vi "DualMotorControl_v0.vi"() -> ()   [LabVIEW 2019]
uses:
  <vilib>/myRIO/Common/Instrument Driver Framework/myRIO v1.0/Encoder/typedefs/Encoder Signal Mode.ctl
  <vilib>/myRIO/Instrument Drivers/Onboard IO/Encoder/typedefs/Encoder Reference.ctl
  <vilib>/myRIO/Common/Instrument Driver Framework/Utilities/typedefs/myRIO Generic Hardware Reference.ctl
  <vilib>/myRIO/Common/Instrument Driver Framework/Utilities/typedefs/Hardware Version Enum.ctl
  <vilib>/myRIO/Common/Instrument Driver Framework/Utilities/typedefs/myRIO v1.0 Reference.ctl
  <vilib>/myRIO/Common/Instrument Driver Framework/Utilities/typedefs/Generic FPGA Reference.ctl
  <vilib>/myRIO/Common/Instrument Driver Framework/myRIO v1.0/Encoder/typedefs/Encoder Channels Enum.ctl
  <vilib>/myRIO/Common/Instrument Driver Framework/myRIO v1.0/Encoder/typedefs/Encoder Configuration v1.0.ctl
  <vilib>/userDefined/High Color/nirio_resource_hc.ctl
  <vilib>/Platform/TimedLoop/XDataNode/timing_clust.ctl
  <vilib>/Platform/TimedLoop/XDataNode/nitl_modes.ctl
  <vilib>/Platform/TimedLoop/XDataNode/wakeup.ctl
  <vilib>/myRIO/Instrument Drivers/Onboard IO/PWM/typedefs/PWM Reference.ctl
  <vilib>/myRIO/Common/Instrument Driver Framework/myRIO v1.0/PWM/typedefs/PWM Channels Enum.ctl
  <vilib>/myRIO/Instrument Drivers/Onboard IO/PWM/typedefs/PWM Configuration.ctl
  <vilib>/myRIO/Instrument Drivers/Onboard IO/DIO/typedefs/DIO Reference.ctl
  <vilib>/myRIO/Common/Instrument Driver Framework/myRIO v1.0/DIO/typedefs/DIO Channels List.ctl
  <vilib>/myRIO/Common/Instrument Driver Framework/myRIO v1.0/DIO/typedefs/DIO Channels Enum.ctl
  <vilib>/myRIO/Common/Instrument Driver Framework/Utilities/vis/Is FPGA Ref Available.vi
  <vilib>/myRIO/Common/Instrument Driver Framework/myRIO v1.0/Encoder/vis/myRIO v1.1 Open Encoder.vi
  <vilib>/myRIO/Instrument Drivers/Onboard IO/Encoder/vis/Read.vi
  <vilib>/myRIO/Common/Instrument Driver Framework/myRIO v1.0/PWM/vis/myRIO v1.1 Open PWM.vi
  <vilib>/myRIO/Instrument Drivers/Onboard IO/PWM/vis/Set Duty Cycle and Frequency.vi
  <vilib>/myRIO/Common/Instrument Driver Framework/myRIO v1.0/DIO/vis/myRIO v1.1 Open DIO.vi
  <vilib>/myRIO/Instrument Drivers/Onboard IO/DIO/vis/Write.vi
  <vilib>/myRIO/Common/Instrument Driver Framework/Utilities/vis/Validate Channels.vi
  <vilib>/myRIO/Common/Instrument Driver Framework/myRIO v1.0/Encoder/vis/myRIO v1.0 Reserve Encoder.vi
  <vilib>/myRIO/Common/Instrument Driver Framework/myRIO v1.0/PWM/vis/myRIO v1.0 Reserve PWM.vi
  <vilib>/myRIO/Common/Instrument Driver Framework/myRIO v1.0/DIO/vis/myRIO v1.0 Reserve DIO.vi
  <vilib>/myRIO/Common/Instrument Driver Framework/myRIO v1.0/Encoder/vis/myRIO v1.0 Build MUX Configuration Encoder.vi
  <vilib>/myRIO/Common/Instrument Driver Framework/myRIO v1.0/Resource Manager/vis/myRIO v1.0 Reserve Channel List.vi
  <vilib>/myRIO/Common/Instrument Driver Framework/myRIO v1.0/PWM/vis/myRIO v1.0 Build MUX Configuration PWM.vi
  <vilib>/myRIO/Common/Instrument Driver Framework/myRIO v1.0/DIO/vis/myRIO v1.0 Build MUX Configuration DIO.vi
  <vilib>/myRIO/Common/Instrument Driver Framework/myRIO v1.0/Resource Manager/vis/myRIO v1.0 Create Configuration List.vi
  <vilib>/myRIO/Common/Instrument Driver Framework/myRIO v1.0/Resource Manager/vis/myRIO v1.0 Reserve Channel.vi
  <vilib>/myRIO/Common/Instrument Driver Framework/myRIO v1.0/Resource Manager/vis/myRIO v1.0 Unreserve Channel.vi
  <vilib>/myRIO/Common/Instrument Driver Framework/myRIO v1.0/Resource Manager/vis/myRIO v1.0 Build Mutex Name.vi
  <vilib>/Utility/VariantDataType/GetNumericInfo.vi
  <vilib>/Utility/error.llb/Error Cluster From Error Code.vi
  <vilib>/myRIO/Common/Instrument Driver Framework/myRIO v1.0/myRIO v1.1 Open.vi
  <vilib>/myRIO/Common/Instrument Driver Framework/Utilities/vis/IO Manager.vi
  <vilib>/myRIO/Common/Instrument Driver Framework/Utilities/vis/Configuration Manager.vi
  <vilib>/myRIO/Common/Instrument Driver Framework/myRIO v1.0/Resource Manager/vis/myRIO v1.0 Configure IO.vi
  <vilib>/myRIO/Common/Instrument Driver Framework/myRIO v1.0/myRIO v1.0 Close.vi
  <vilib>/myRIO/Common/Instrument Driver Framework/myRIO v1.0/Encoder/vis/myRIO v1.0 Configure Encoder.vi
  <vilib>/myRIO/Common/Instrument Driver Framework/myRIO v1.0/Encoder/vis/myRIO v1.0 Read Encoder.vi
  <vilib>/Instr/_visa.llb/VISA Configure Serial Port (Instr).vi
  <vilib>/myRIO/Common/Instrument Driver Framework/myRIO v1.0/PWM/vis/myRIO v1.0 Write PWM.vi
  <vilib>/myRIO/Common/Instrument Driver Framework/myRIO v1.0/DIO/vis/myRIO v1.0 Write DIO.vi
  <vilib>/Utility/file.llb/Write Delimited Spreadsheet (DBL).vi
  <vilib>/myRIO/Express VI/Onboard IO/Encoder/Encoder Express VI.xnode
  <vilib>/myRIO/Instrument Drivers/Onboard IO/Encoder/vis/myRIO Encoder Open.xnode
  <vilib>/myRIO/Common/Instrument Driver Framework/myRIO v1.0/Encoder/typedefs/Encoder Count Direction Enum.ctl
  <vilib>/platform/TimedLoop/XDataNode/XDataNode.xnode
  <vilib>/myRIO/Express VI/Onboard IO/PWM/PWM Express VI.xnode
  <vilib>/myRIO/Instrument Drivers/Onboard IO/PWM/vis/myRIO PWM Open.xnode
  <vilib>/myRIO/Express VI/Onboard IO/DO/DO Express VI.xnode
  <vilib>/myRIO/Instrument Drivers/Onboard IO/DIO/vis/myRIO DIO Open.xnode
  <vilib>/Platform/TimedLoop/XDataNode/XDNodeRunTimeDep.lvlib
  <vilib>/myRIO/Instrument Drivers/Onboard IO/Encoder/Encoder.lvlib
  <vilib>/myRIO/Instrument Drivers/Onboard IO/DIO/DIO.lvlib
  <vilib>/myRIO/Instrument Drivers/Onboard IO/PWM/PWM.lvlib
panel:
  out "DC Velocity Graph":cluster{dbl[], dbl[]}[](graph)
  out "DC Position Graph":cluster{dbl[], dbl[]}[](graph)
  out "DC Velocity Chart":cluster{dbl, dbl}(graph)
  out "Duty cycle":dbl(graph)
  out "Duty cycle":dbl
  in  "Frequency":dbl=1000.0
  in  "Gain":T1={"P Gain"=0.5, "I Gain"=0.0, "D Gain"=0.005}
  out "DC Position Chart":cluster{dbl, dbl}(graph)
  in  "Encoder_Count":dbl=54991.0
  in  "t_shift":dbl=0.000125
  in  "T_ratio":dbl=10.0
  in  "buffer ratio":dbl=0.3
  in  "first or second tripod":bool
  in  "data of 5th order formula\nts,tair,a1-a6":dbl[](array[numeric])
  in  "format (%.3f)":string="%.3f"
  in  "file path (dialog if empty)":path
  out "error out":errorcluster
  in  "baud rate (9600)":u32=500000
  in  "VISA resource name":refnum<visa-resource-name>="ASRL2::INSTR"
  in  "stop":bool
  in  "const posotion":dbl=180.0
  out "write to visa":string
  out "read from visa":string
  out "sine position":dbl
  out "time":dbl
  out "iteration":i32
  in  "const(f)/sine(t)":bool
  in  "graph plot freq.":i32=1
  out "Servo Position Graph":cluster{dbl[], dbl[]}[](graph)
  in  "sinewave period":dbl=10.0
  in  "Loop Period":i64=5
  # "Servo motor"
  # "Read data to csv file"
  # "Read data to csv file"
  # "visa setting"
  # "servo setting"
  # "Timed loop status"
  # "DC motor"
  # "R-SLIP Parameters"
  # "v = 1; a = 15"
  # "v = 1.25; a = 15"
  # "v = 1.5; a = 15"
  # "0.184067181524967\n0.263820978418769\n256152.551336786\n-30272.30000274\n-9876.03760433421\n-1096.38594197941\n885.91817900106\n-44.6781799901984"
  # "0.215241998794118\n0.254514142390288\n4771.41078363533\n62185.8763006578\n-22508.5336527453\n390.805502041188\n686.695311017595\n-40.4128145310291"
  # "0.163616269216122\n0.27489641502463\n771965.39318528\n-201617.027694185\n8828.08396944145\n-2683.04589908678\n1085.57303422127\n-48.5860395324432"
  # "v = 1.75; a = 15"
  # "v = 2; a = 15"
  # "v = 2.25; a = 15"
  # "0.148651048423414\n0.288542414074344\n1776973.44893281\n-511591.467559457\n38775.9830765103\n-4576.94506688942\n1289.39828252671\n-52.3115561007577"
  # "0.136976185169818\n0.304016701267508\n3461279.85083822\n-993110.73746345\n80544.6579529191\n-6699.48295844177\n1494.82265451498\n-55.8934424469099"
  # "0.134381902205816\n0.369022171779704\n3272804.8365432\n-899365.569589567\n71225.2463409934\n-7039.10791102172\n1512.66147498591\n-59.3408899720725"
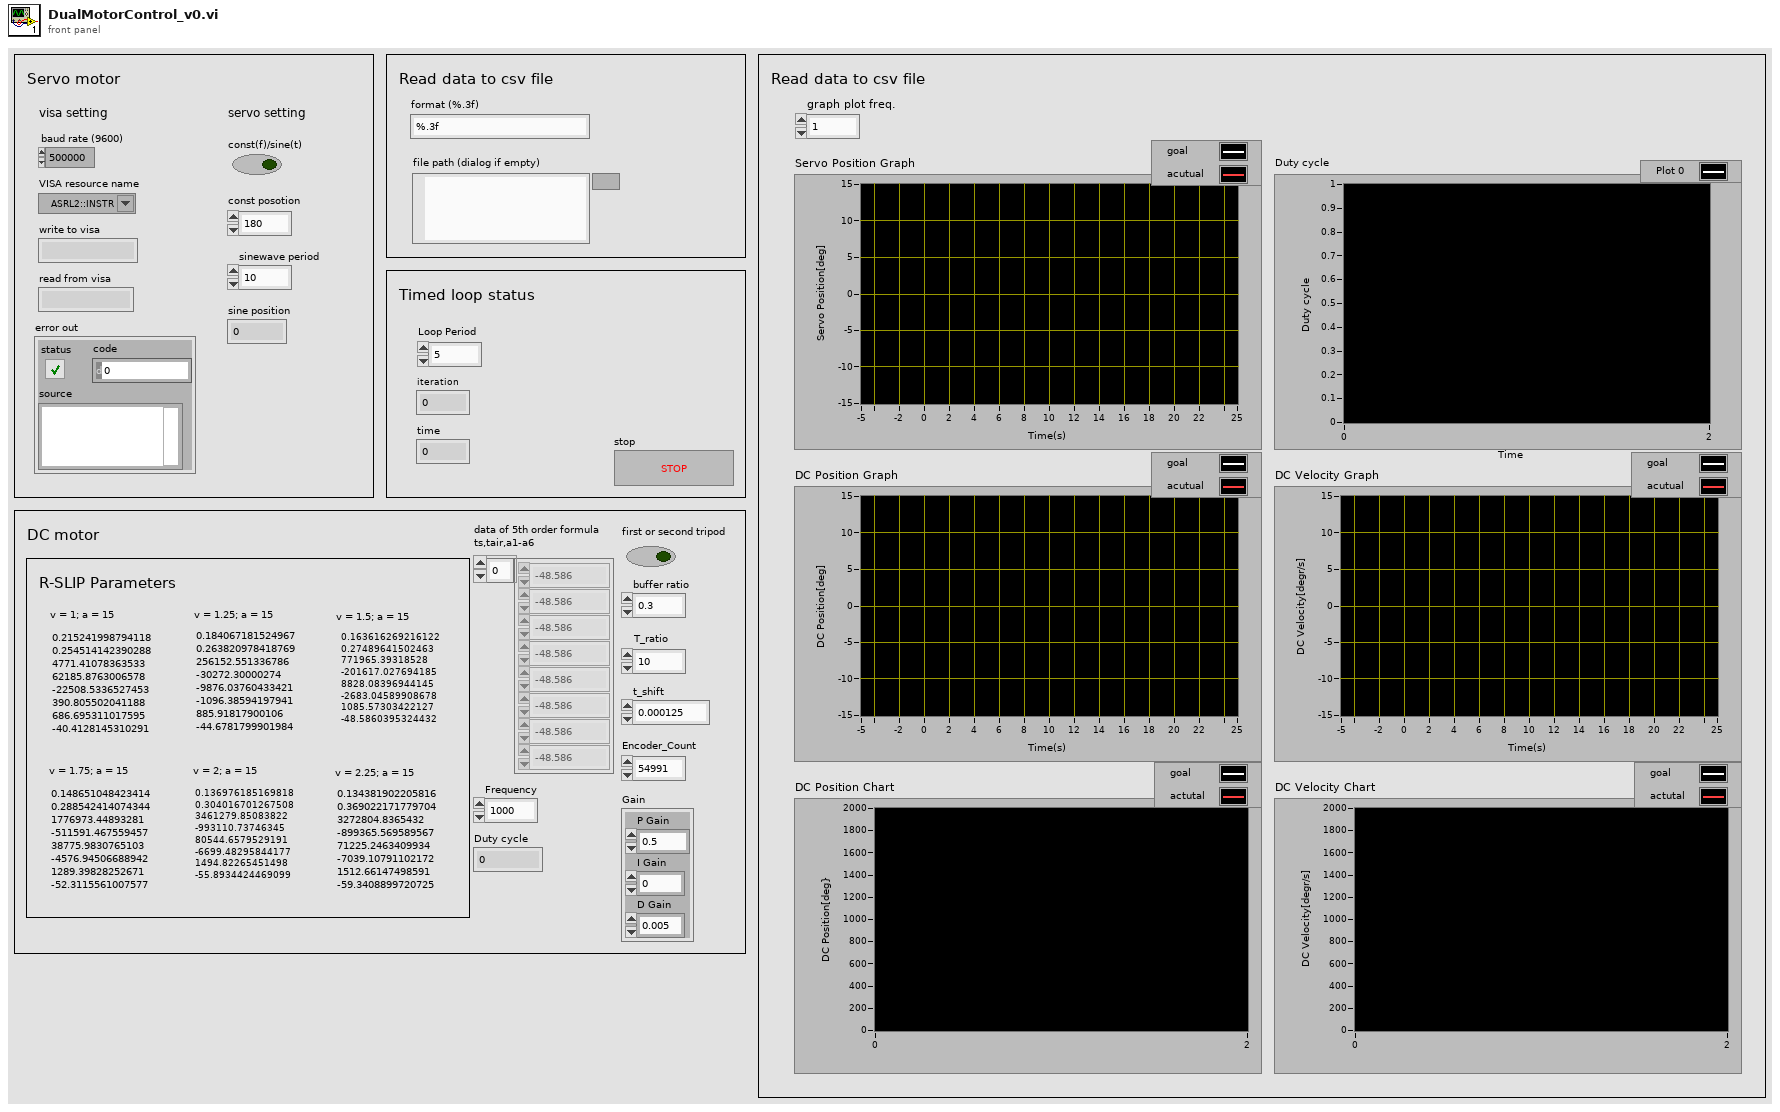
[diagram p1: front panel]
types:
  T1 = cluster{"P Gain":dbl, "I Gain":dbl, "D Gain":dbl}
  T2 = typedef "Encoder.lvlib/Encoder Reference.ctl" = cluster{"myRIO Reference":T3, "Encoder Channels Enum":T7}
  T3 = typedef "myRIO Generic Hardware Reference.ctl" = cluster{"myRIO Model":T4, "myRIO Hardware Reference":T5}
  T4 = typedef "Hardware Version Enum.ctl" = enum16{"Unknown", "myRIO-1900", "myRIO-1950", "roboRIO", "NI ELVIS RIO CM", "ELVIS III"}
  T5 = typedef "myRIO v1.0 Reference.ctl" = cluster{"Generic FPGA Reference":T6, "Allow multiple opens":bool}
  T6 = typedef "Generic FPGA Reference.ctl" = refnum<k20>
  T7 = typedef "Encoder Channels Enum.ctl" = enum16{"Not Connected", "C/ENC0", "C/ENC1", "A/ENC", "A/ENC0", "A/ENC1", "A/ENC2", "A/ENC3", "A/ENC4", "A/ENC5", "A/ENC6", "A/ENC7", "A/ENC8", "A/ENC9", "B/ENC", "B/ENC0", "B/ENC1", "B/ENC2", "B/ENC3", "B/ENC4", "B/ENC5", "B/ENC6", "B/ENC7", "B/ENC8", "B/ENC9", "DIO/ENC0", "DIO/ENC1", "DIO/ENC2", "DIO/ENC3", "DIO/ENC4"}
  T8 = typedef "Encoder Signal Mode.ctl" = enum16{"Quadrature phase signal", "Step and direction signal"}
  T9 = typedef "nirio_resource_hc.ctl" = tag
  T10 = cluster{"set position":dbl, "set position":dbl, "set position":dbl, "set position":dbl, "set position":dbl, "set position":dbl}
  T11 = typedef "DIO.lvlib/DIO Reference.ctl" = cluster{"myRIO Reference":T3, "DIO Channels List":T12}
  T12 = typedef "DIO Channels List.ctl" = T13[]
  T13 = typedef "DIO Channels Enum.ctl" = enum16{"Not Connected", "C/DIO0", "C/DIO1", "C/DIO2", "C/DIO3", "C/DIO4", "C/DIO5", "C/DIO6", "C/DIO7", "A/DIO0", "A/DIO1", "A/DIO2", "A/DIO3", "A/DIO4", "A/DIO5", "A/DIO6", "A/DIO7", "A/DIO8", "A/DIO9", "A/DIO10", "A/DIO11", "A/DIO12", "A/DIO13", "A/DIO14", "A/DIO15", "A/DIO16", "A/DIO17", "A/DIO18", "A/DIO19", "B/DIO0", "B/DIO1", "B/DIO2", "B/DIO3", "B/DIO4", "B/DIO5", "B/DIO6", "B/DIO7", "B/DIO8", "B/DIO9", "B/DIO10", "B/DIO11", "B/DIO12", "B/DIO13", "B/DIO14", "B/DIO15", "B/DIO16", "B/DIO17", "B/DIO18", "B/DIO19", "LED0", "LED1", "LED2", "LED3", "Button0", "DIO/DIO0", "DIO/DIO1", "DIO/DIO2", "DIO/DIO3", "DIO/DIO4", "DIO/DIO5", "DIO/DIO6", "DIO/DIO7", "DIO/DIO8", "DIO/DIO9", "SPI/CS0", "SPI/CS1", "SPI/CS2", "SPI/CS3", "LED RADIO (Green)", "LED RADIO (Red)", "LED COMM (Green)", "LED COMM (Red)", "LED MODE (Green)", "LED MODE (Red)"}
  T14 = typedef "PWM.lvlib/PWM Reference.ctl" = cluster{"myRIO Reference":T3, "PWM Channels Enum":T15, "PWM Configuration":T16}
  T15 = typedef "PWM Channels Enum.ctl" = enum16{"Not Connected", "C/PWM0", "C/PWM1", "A/PWM0", "A/PWM1", "A/PWM2", "A/PWM3", "A/PWM4", "A/PWM5", "A/PWM6", "A/PWM7", "A/PWM8", "A/PWM9", "A/PWM10", "A/PWM11", "A/PWM12", "A/PWM13", "A/PWM14", "A/PWM15", "A/PWM16", "A/PWM17", "A/PWM18", "A/PWM19", "B/PWM0", "B/PWM1", "B/PWM2", "B/PWM3", "B/PWM4", "B/PWM5", "B/PWM6", "B/PWM7", "B/PWM8", "B/PWM9", "B/PWM10", "B/PWM11", "B/PWM12", "B/PWM13", "B/PWM14", "B/PWM15", "B/PWM16", "B/PWM17", "B/PWM18", "B/PWM19", "PWM/PWM0", "PWM/PWM1", "PWM/PWM2", "PWM/PWM3", "PWM/PWM4", "PWM/PWM5", "PWM/PWM6", "PWM/PWM7", "PWM/PWM8", "PWM/PWM9"}
  T16 = typedef "PWM.lvlib/PWM Configuration.ctl" = cluster{"Frequency":dbl, "Duty Cycle":dbl}
  T17 = typedef "XDNodeRunTimeDep.lvlib/timing_clust.ctl" = cluster{"Expected End [f-1]":u64, "Actual End [f-1]":u64, "Finished Late? [f-1]":bool, "Expected End [i-1]":u64, "Actual End [i-1]":u64, "Finished Late? [i-1]":bool, "Expected Start [i]":u64, "Actual Start [i]":u64, "Expected Start [f]":u64, "Actual Start [f]":u64, "Source Name":string, "Structure Name":string, "Period":i64, "Deadline":i64, "Offset":i64, "Start":i64, "Priority":i32, "Timeout":i32, "Mode":T18, "Wakeup Reason":T19, "Error":errorcluster, "Source Type":string, "Secondary Source Type":string, "Global End Time":u64, "Global Start Time":u64, "Frame Duration":u64, "Iteration Duration":u64, "Assigned CPU":i32, "I/O Scan Engine Mode":u32}
  T18 = typedef "XDNodeRunTimeDep.lvlib/nitl_modes.ctl" = enum32{"No Change", "Process missed periods, maintain original phase", "Discard missed periods, maintain original phase", "Process missed periods, ignore original phase", "Discard missed periods, ignore original phase"}
  T19 = typedef "XDNodeRunTimeDep.lvlib/wakeup.ctl" = enum32{"Normal", "Aborted", "Asynchronous wakeup", "Timing source error", "Timed loop error", "Timeout"}
  T20 = cluster{"[0]":dbl, "[1]":dbl, "[2]":dbl, "[3]":dbl, "[4]":dbl, "[5]":dbl}
  T21 = cluster{"set position":i32, "set position":i32, "set position":i32, "set position":i32, "set position":i32, "set position":i32}
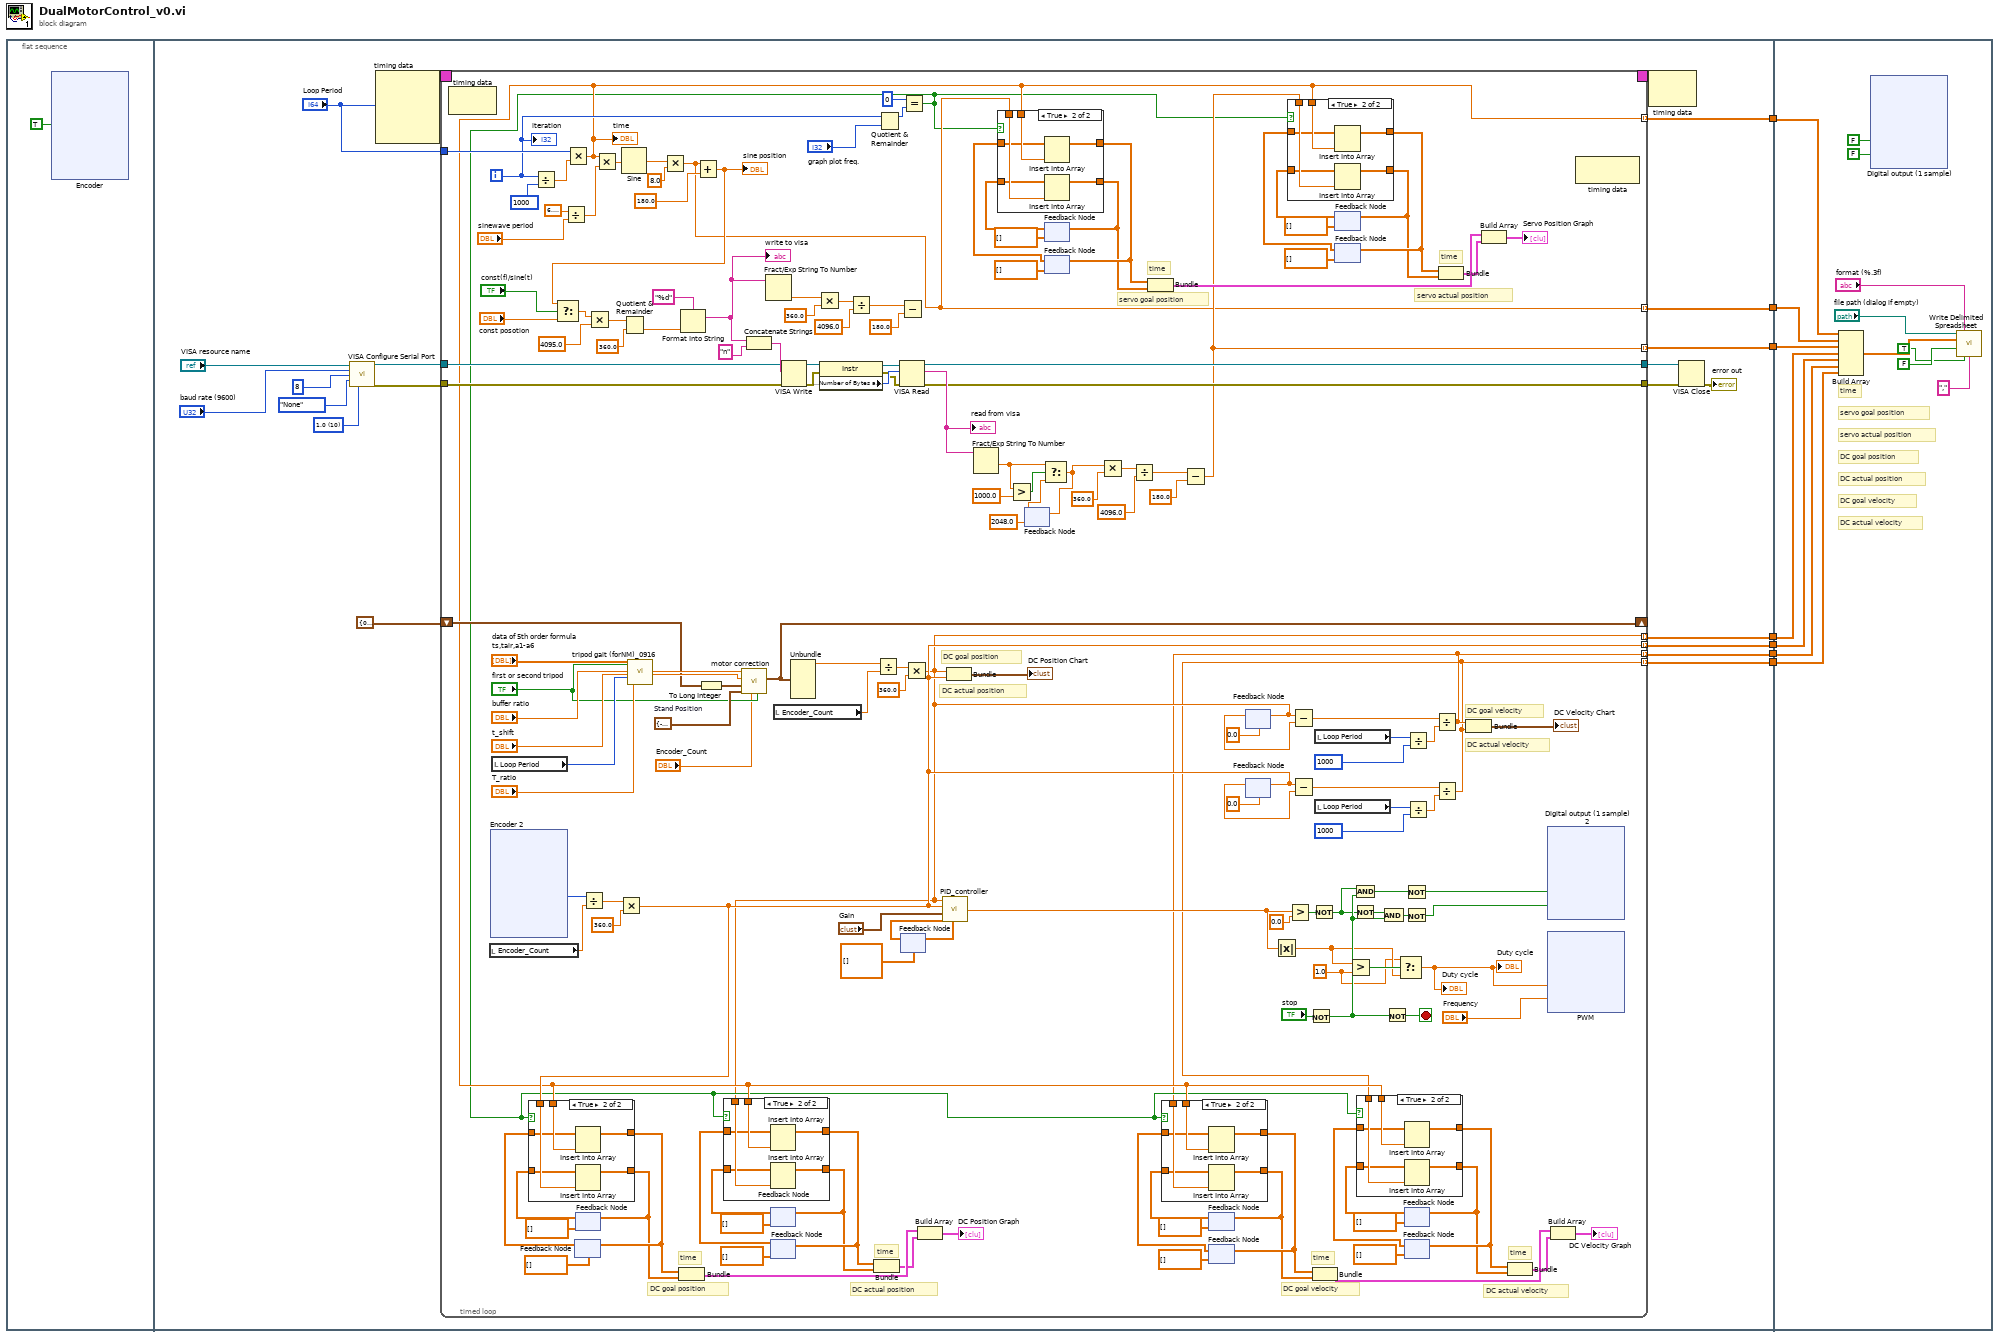
[diagram p0: block diagram]
diagram:
  n1 = flat-sequence {
    tunnel: [w63] -> w7
    tunnel: [w62] -> w6
    tunnel: [w61] -> w5
    tunnel: [w59] -> w4
    tunnel: [w58] -> w3
    tunnel: [w57] -> w2
    tunnel: [w56] -> w1
    tunnel: w7 -> [w414]
    tunnel: w6 -> [w413]
    tunnel: w5 -> [w415]
    tunnel: w4 -> [w412]
    tunnel: w3 -> [w411]
    tunnel: w2 -> [w410]
    tunnel: w1 -> [w409]
    frame #0 {
      n2 = xnode "Encoder"("Reset Counter"=TRUE) -> ()  [unwired: 1 in, 4 out]
    }
    frame #1 {
      w70 = u16 10 items=["1.0"=10, "1.5"=15, "2.0"=20] ("stop bits (10: 1 bit)")
      n3 = call-poly "VISA Configure Serial Port"("VISA resource name"="VISA resource name", "baud rate (9600)"="baud rate (9600)", "data bits (8)"=u16 8, "parity (0:none)"=enum16{"None", "Odd", "Even", "Mark", "Space"}."None", "stop bits (10: 1 bit)"=w70) -> ("VISA resource name out"=w69:refnum<visa-resource-name>, "error out"=w68:errorcluster)  [unwired: 9 in]
      n4 = node-c288("Loop Period") -> (w75:T17)  [unwired: 3 in]
      n5 = timed-loop {
        timing: w75 -> [_]
        timing-out: [_] -> w74
        tunnel: "Loop Period" -> [w184]
        tunnel: w68 -> [w185]
        tunnel: [w182] -> w67
        tunnel: w69 -> [w186]
        tunnel: [w181] -> w60
        tunnel: [w99] -> w63 mode=indexing
        tunnel: [w180] -> w62 mode=indexing
        tunnel: [w80] -> w61 mode=indexing
        shift-right: [w161] -> _
        shift-left: T10 {"set position"=0.0, "set position"=0.0, "set position"=0.0, "set position"=0.0, "set position"=0.0, "set position"=0.0} ("Setpoint_to_motor") -> [w162]
        tunnel: [w78] -> w59 mode=indexing
        tunnel: [w96] -> w58 mode=indexing
        tunnel: [w77] -> w57 mode=indexing
        tunnel: [w76] -> w56 mode=indexing
        i -> [w183]
        stop <- w131 stop-if-true
        w128 = 1.0 ("y")
        w160 = T20 {"[0]"=-27495.5, "[1]"=-27495.5, "[2]"=-27495.5, "[3]"=-27495.5, "[4]"=-27495.5, "[5]"=-27495.5}  # Stand Position
        # "time"
        # "DC actual velocity"
        # "time"
        # "DC goal velocity"
        # "time"
        # "DC actual position"
        # "time"
        # "DC goal position"
        # "DC actual velocity"
        # "DC goal velocity"
        # "DC actual position"
        # "DC goal position"
        # "time"
        # "servo actual position"
        # "time"
        # "servo goal position"
        n6 = node-c288() -> ()  [unwired: 1 in, 1 out]
        n7 = local read "Encoder_Count"() -> (w153:dbl)
        n8 = xnode "Encoder 2"() -> ("Counter Value"=w152:i32)  [unwired: 2 in, 3 out]
        n9 = local read "Loop Period"() -> (w167:i64)
        n10 = Divide(x=w183, y=i64 1000) -> (x/y=w216:dbl)
        n11 = Divide(x=6.283185307179586, y="sinewave period") -> (x/y=w171:dbl)
        n12 = Multiply(x=w184, y=w216) -> (x*y=w80:dbl)
        "time" <- w80
        n13 = feedback #1(dbl[] []) -> (w111:dbl[])
        n14 = feedback #2(dbl[] []) -> (w114:dbl[])
        n15 = Divide(x=w152, y=w153) -> (x/y=w150:dbl)
        n16 = Multiply(x=w80, y=w171) -> (x*y=w219:dbl)
        n17 = Multiply(x=w150, y=360.0 ("x")) -> (x*y=w96:dbl)
        n18 = Sine(x=w219) -> (sin(x)=w204:dbl)
        n19 = call "tripod gait (forNM)_0916.vi"("data of 5th order formula\nts,tair,a1-a6"="data of 5th order formula\nts,tair,a1-a6", "first or second"="first or second tripod", "buffer ratio"="buffer ratio", "t_shift"="t_shift", "sample time"=w167, "T_ratio"="T_ratio") -> ("Set Point"=w165:dbl, "Set Point 2"=w164:dbl)  [unwired: 4 in, 16 out]
        n20 = Multiply(x=w204, y=8.0) -> (x*y=w99:dbl)
        n21 = Add(x=w99, y=180.0) -> (x+y=w214:dbl)
        "sine position" <- w214
        n22 = Select(t=w214, s="const(f)/sine(t)", f="const posotion") -> (s? t:f=w212:dbl)
        n23 = Multiply(x=w212, y=4095.0) -> (x*y=w235:dbl)
        n24 = Quotient & Remainder(x=w235, y=360.0) -> (floor(x/y)=w233:dbl)  [unwired: 1 out]
        n25 = Format Into String(format string="%d", w233) -> (resulting string=w226:string)  [unwired: 2 in, 1 out]
        "write to visa" <- w226
        n26 = To Long Integer(number=w162) -> (32bit integer=w163:T21)
        n27 = call "motor correction.vi"("first or second"="first or second tripod", "Encoder_Count"="Encoder_Count", "Stand Position"=w160, "encoder position"=w163, "set position 2"=w164, "set position"=w165) -> ("Setpoint_to_motor"=w161:T10)  [unwired: 4 in, 1 out]
        n28 = Concatenate Strings(w226, "n" ("string")) -> (w237:string)
        n29 = Fract/Exp String To Number(string=w226) -> (number=w225:dbl)  [unwired: 3 in, 1 out]
        n30 = feedback #3(dbl[] []) -> (w110:dbl[])
        n31 = feedback #4(dbl[] []) -> (w107:dbl[])
        n32 = local read "Encoder_Count"() -> (w156:dbl)
        n33 = VISA Write(VISA resource name=w186, write buffer=w237, error in (no error)=w185) -> (VISA resource name out=w202:refnum<visa-resource-name>, error out=w201:errorcluster)  [unwired: 1 out]
        n34 = Unbundle(w161) -> ("set position"=w158:dbl)  [unwired: 5 out]
        n35 = Multiply(x=w225, y=360.0 ("x")) -> (x*y=w223:dbl)
        n36 = property class="Instr"(reference=w202, error in=w201) -> (reference out=w199:refnum<visa-resource-name>, error out=w198:errorcluster, "Serial Settings:Number of Bytes at Serial Port"=w200:u32)
        n37 = Divide(x=w223, y=4096.0) -> (x/y=w228:dbl)
        n38 = Divide(x=w158, y=w156) -> (x/y=w155:dbl)
        n39 = Quotient & Remainder(x=w183, y="graph plot freq.") -> (x-y*floor(x/y)=w207:i32)  [unwired: 1 out]
        n40 = VISA Read(VISA resource name=w199, byte count=w200, error in (no error)=w198) -> (VISA resource name out=w181:refnum<visa-resource-name>, read buffer=w227:string, error out=w182:errorcluster)  [unwired: 1 out]
        "read from visa" <- w227
        n41 = Subtract(x=w228, y=180.0) -> ()  [unwired: 1 out]
        n42 = feedback #5(dbl[] [] ("state(k)")) -> (w147:dbl[])
        n43 = Equal?(x=0, y=w207) -> (x = y?=w79:bool)
        n44 = case shown="True" w79 {
          tunnel: w80 -> [_ w269]
          tunnel: w96 -> [_ w268]
          tunnel: [w263 w267] -> w97
          tunnel: w114 -> [w263 w266]
          tunnel: [w262 w265] -> w98
          tunnel: w111 -> [w262 w264]
          frame False {
          }
          frame True {
            n45 = Insert Into Array(array=w264, new element=w269) -> (w265:dbl[])  [unwired: 1 in]
            n46 = Insert Into Array(array=w266, new element=w268) -> (w267:dbl[])  [unwired: 1 in]
          }
        }
        n47 = feedback-in #1(w98) -> ()
        n48 = feedback-in #2(w97) -> ()
        n49 = Bundle(w98, w97) -> (w106:cluster{dbl[], dbl[]})  [unwired: 1 in]
        n50 = Multiply(x=w155, y=360.0 ("x")) -> (x*y=w78:dbl)
        n51 = case shown="True" w79 {
          tunnel: w80 -> [_ w261]
          tunnel: w78 -> [_ w260]
          tunnel: [w255 w259] -> w102
          tunnel: w110 -> [w255 w258]
          tunnel: [w254 w257] -> w103
          tunnel: w107 -> [w254 w256]
          frame False {
          }
          frame True {
            n52 = Insert Into Array(array=w256, new element=w261) -> (w257:dbl[])  [unwired: 1 in]
            n53 = Insert Into Array(array=w258, new element=w260) -> (w259:dbl[])  [unwired: 1 in]
          }
        }
        n54 = feedback-in #3(w102) -> ()
        n55 = feedback-in #4(w103) -> ()
        n56 = Bundle(w103, w102) -> (w105:cluster{dbl[], dbl[]})  [unwired: 1 in]
        n57 = Build Array(w106, w105) -> (→"DC Position Graph":cluster{dbl[], dbl[]}[])
        n58 = call "PID_controller.vi"("state(k-1)"=w147, "Gain"="Gain", "variable"=w96, "set point"=w78) -> ("PID gain"=w129:dbl, "state(k)"=w146:dbl[])  [unwired: 1 in]
        n59 = feedback-in #5(w146) -> ()
        n60 = Bundle(w78, w96) -> (→"DC Position Chart":cluster{dbl, dbl})  [unwired: 1 in]
        n61 = Fract/Exp String To Number(string=w227) -> (number=w197:dbl)  [unwired: 3 in, 1 out]
        n62 = Greater?(x=w197, y=1000.0) -> (0:w196:bool)
        n63 = feedback #6(2048.0) -> (w175:dbl)
        n64 = Select(t=w197, s=w196, f=w175) -> (s? t:f=w176:dbl)
        n65 = feedback-in #6(w176) -> ()
        n66 = feedback #7(dbl[] []) -> (w211:dbl[])
        n67 = feedback #8(dbl[] []) -> (w208:dbl[])
        n68 = case shown="True" w79 {
          tunnel: w80 -> [_ w402]
          tunnel: w99 -> [_ w401]
          tunnel: [w396 w400] -> w100
          tunnel: w211 -> [w396 w399]
          tunnel: [w395 w398] -> w101
          tunnel: w208 -> [w395 w397]
          frame False {
          }
          frame True {
            n69 = Insert Into Array(array=w397, new element=w402) -> (w398:dbl[])  [unwired: 1 in]
            n70 = Insert Into Array(array=w399, new element=w401) -> (w400:dbl[])  [unwired: 1 in]
          }
        }
        n71 = feedback-in #7(w100) -> ()
        n72 = feedback-in #8(w101) -> ()
        n73 = Multiply(x=w176, y=360.0 ("x")) -> (x*y=w220:dbl)
        n74 = Divide(x=w220, y=4096.0) -> (x/y=w222:dbl)
        n75 = Bundle(w101, w100) -> (w191:cluster{dbl[], dbl[]})  [unwired: 1 in]
        n76 = Subtract(x=w222, y=180.0) -> (x-y=w180:dbl)
        n77 = feedback #9(dbl[] []) -> (w95:dbl[])
        n78 = feedback #10(dbl[] []) -> (w92:dbl[])
        n79 = feedback #11(0.0) -> (w122:dbl)
        n80 = feedback-in #11(w78) -> ()
        n81 = feedback #12(0.0) -> (w116:dbl)
        n82 = feedback-in #12(w96) -> ()
        n83 = Absolute Value(x=w129) -> (abs(x)=w138:dbl)
        n84 = Greater?(x=w129, y=0.0) -> (0:w140:bool)
        n85 = Subtract(x=w78, y=w122) -> (x-y=w125:dbl)
        n86 = Subtract(x=w96, y=w116) -> (x-y=w118:dbl)
        n87 = Not(x="stop") -> (.not. x?=w142:bool)
        n88 = Not(x=w140) -> (.not. x?=w137:bool)
        n89 = local read "Loop Period"() -> (w124:i64)
        n90 = local read "Loop Period"() -> (w115:i64)
        n91 = feedback #13(dbl[] []) -> (w195:dbl[])
        n92 = feedback #14(dbl[] []) -> (w192:dbl[])
        n93 = case shown="True" w79 {
          tunnel: w80 -> [_ w394]
          tunnel: w180 -> [_ w393]
          tunnel: [w388 w392] -> w187
          tunnel: w195 -> [w388 w391]
          tunnel: [w387 w390] -> w188
          tunnel: w192 -> [w387 w389]
          frame False {
          }
          frame True {
            n94 = Insert Into Array(array=w389, new element=w394) -> (w390:dbl[])  [unwired: 1 in]
            n95 = Insert Into Array(array=w391, new element=w393) -> (w392:dbl[])  [unwired: 1 in]
          }
        }
        n96 = feedback-in #13(w187) -> ()
        n97 = feedback-in #14(w188) -> ()
        n98 = Greater?(x=w138, y=w128) -> (0:w139:bool)
        n99 = And(x=w137, y=w142) -> (x .and. y?=w134:bool)
        n100 = Not(x=w137) -> (.not. x?=w143:bool)
        n101 = And(x=w143, y=w142) -> (x .and. y?=w136:bool)
        n102 = Not(x=w142) -> (.not. x?=w131:bool)
        n103 = Select(t=w128, s=w139, f=w138) -> (s? t:f=w132:dbl)
        "Duty cycle" <- w132
        "Duty cycle" <- w132
        n104 = Not(x=w134) -> (.not. x?=w133:bool)
        n105 = Not(x=w136) -> (.not. x?=w135:bool)
        n106 = feedback #15(dbl[] []) -> (w91:dbl[])
        n107 = feedback #16(dbl[] []) -> (w88:dbl[])
        n108 = Divide(x=w124, y=i64 1000) -> (x/y=w126:dbl)
        n109 = Divide(x=w115, y=i64 1000) -> (x/y=w119:dbl)
        n110 = Divide(x=w125, y=w126) -> (x/y=w77:dbl)
        n111 = case shown="True" w79 {
          tunnel: w80 -> [_ w253]
          tunnel: w77 -> [_ w252]
          tunnel: [w247 w251] -> w81
          tunnel: w95 -> [w247 w250]
          tunnel: [w246 w249] -> w82
          tunnel: w92 -> [w246 w248]
          frame False {
          }
          frame True {
            n112 = Insert Into Array(array=w248, new element=w253) -> (w249:dbl[])  [unwired: 1 in]
            n113 = Insert Into Array(array=w250, new element=w252) -> (w251:dbl[])  [unwired: 1 in]
          }
        }
        n114 = feedback-in #9(w81) -> ()
        n115 = feedback-in #10(w82) -> ()
        n116 = Bundle(w82, w81) -> (w87:cluster{dbl[], dbl[]})  [unwired: 1 in]
        n117 = Divide(x=w118, y=w119) -> (x/y=w76:dbl)
        n118 = case shown="True" w79 {
          tunnel: w80 -> [_ w245]
          tunnel: w76 -> [_ w244]
          tunnel: [w239 w243] -> w83
          tunnel: w91 -> [w239 w242]
          tunnel: [w238 w241] -> w84
          tunnel: w88 -> [w238 w240]
          frame False {
          }
          frame True {
            n119 = Insert Into Array(array=w240, new element=w245) -> (w241:dbl[])  [unwired: 1 in]
            n120 = Insert Into Array(array=w242, new element=w244) -> (w243:dbl[])  [unwired: 1 in]
          }
        }
        n121 = feedback-in #15(w83) -> ()
        n122 = feedback-in #16(w84) -> ()
        n123 = Bundle(w188, w187) -> (w190:cluster{dbl[], dbl[]})  [unwired: 1 in]
        n124 = Bundle(w77, w76) -> (→"DC Velocity Chart":cluster{dbl, dbl})  [unwired: 1 in]
        n125 = Build Array(w191, w190) -> (→"Servo Position Graph":cluster{dbl[], dbl[]}[])
        n126 = Bundle(w84, w83) -> (w86:cluster{dbl[], dbl[]})  [unwired: 1 in]
        n127 = xnode "Digital output (1 sample) 2"("A/DIO0 (Pin 11)"=w133, "A/DIO1 (Pin 13)"=w135) -> ()  [unwired: 1 in, 1 out]
        n128 = xnode "PWM"("Duty Cycle"=w132, "Frequency [Hz]"="Frequency") -> ()  [unwired: 1 in, 1 out]
        n129 = Build Array(w87, w86) -> (→"DC Velocity Graph":cluster{dbl[], dbl[]}[])
        n130 = node-c288() -> ()  [unwired: 1 in, 1 out]
        "iteration" <- w183
      }
      n131 = node-c288(w74) -> ()  [unwired: 1 out]
      n132 = VISA Close(VISA resource name=w60, error in (no error)=w67) -> (error out=→"error out":errorcluster)
    }
    frame #2 {
      # "DC actual velocity"
      # "DC goal velocity"
      # "DC actual position"
      # "DC goal position"
      # "time"
      # "servo actual position"
      # "servo goal position"
      n133 = Build Array(w415, w414, w413, w412, w411, w410, w409) -> (w421:dbl[][])
      n134 = xnode "Digital output (1 sample)"("A/DIO0 (Pin 11)"=FALSE, "A/DIO1 (Pin 13)"=FALSE) -> ()  [unwired: 1 in, 1 out]
      n135 = call-poly <vilib>:"Write Delimited Spreadsheet.vi"("file path (dialog if empty)"="file path (dialog if empty)", "format (%.3f)"="format (%.3f)", "2D data"=w421, "append to file? (new file:F)"=FALSE ("transpose? (no:F)"), "transpose? (no:F)"=TRUE ("append to file? (new file:F)"), "delimiter (\\t)"="," ("delimiter (\\t)")) -> ()  [unwired: 8 in, 2 out]
    }
  }
